vi "IDS Set Get ROI.vi"(0 "IDS Notifier Ref":refnum<notifier>, 5 "IDS Actions":T1, 7 "IDS Camera Ref":refnum<k24>, 9 "IDS Image Ref":T2, 11 "Error":errorcluster) -> (4 "IDS Notifier Ref (Dup)":refnum<notifier>, 15 "Error":errorcluster)   [LabVIEW 2025]
uses:
  C:/Users/Photonics03/Documents/Microscope-Control/Device Library/Cameras/IDS/IDS LabView Examples/LabVIEW/ueye.NET/uEyeDotNet.dll
  IDS LabView Examples/LabVIEW/ueye.NET/uEyeDotNet.dll
  <vilib>/vision/Image Controls.llb/IMAQ Image.ctl
  IDS Controls/IDS Notifier Element.ctl
  IDS Controls/IDS Actions.ctl
  IDS Controls/IDS Parameters.ctl
  IDS Controls/IDS Parameter List.ctl
  IDS Controls/IDS ROI.ctl
  Camera Controls/Camera IMAQ Key Info.ctl
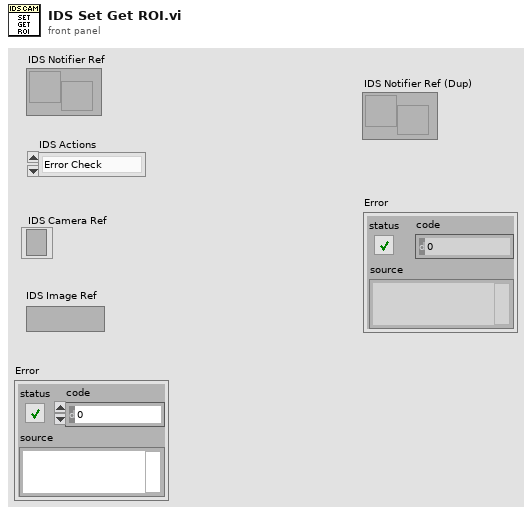
[diagram p1: front panel]
types:
  T1 = typedef "IDS Actions.ctl" = enum16{"Error Check", "Initialize", "Preview", "Record", "Abort", "Record Settings", "Set Parameter", "Get Parameter", "Set ROI", "Get ROI", "Status", "Quit"}
  T2 = typedef "IMAQ Image.ctl" = refnum<image>
  T3 = typedef "Camera IMAQ Key Info.ctl" = cluster{"Frame":u32, "Sensor Height":i32, "Sensor Width":i32, "ROI Height":i32, "ROI Width":i32, "ROI Enable?":bool, "Bit per Pixel":u8}
  T4 = typedef "IDS Notifier Element.ctl" = cluster{"IDS Actions":T1, "Received?":bool, "IDS Parameter":T5, "IDS ROI":T7, "Running?":bool, "File Path":path, "# of frames":u32, "Image Ref":T2, "Error":errorcluster, "Binning":i32}
  T5 = typedef "IDS Parameters.ctl" = cluster{"Parameter":T6, "Value":dbl}
  T6 = typedef "IDS Parameter List.ctl" = enum16{"Exposure Time (s)", "Binning"}
  T7 = typedef "IDS ROI.ctl" = cluster{"H Offset":i32, "V Offset":i32, "H Width":i32, "V Width":i32}
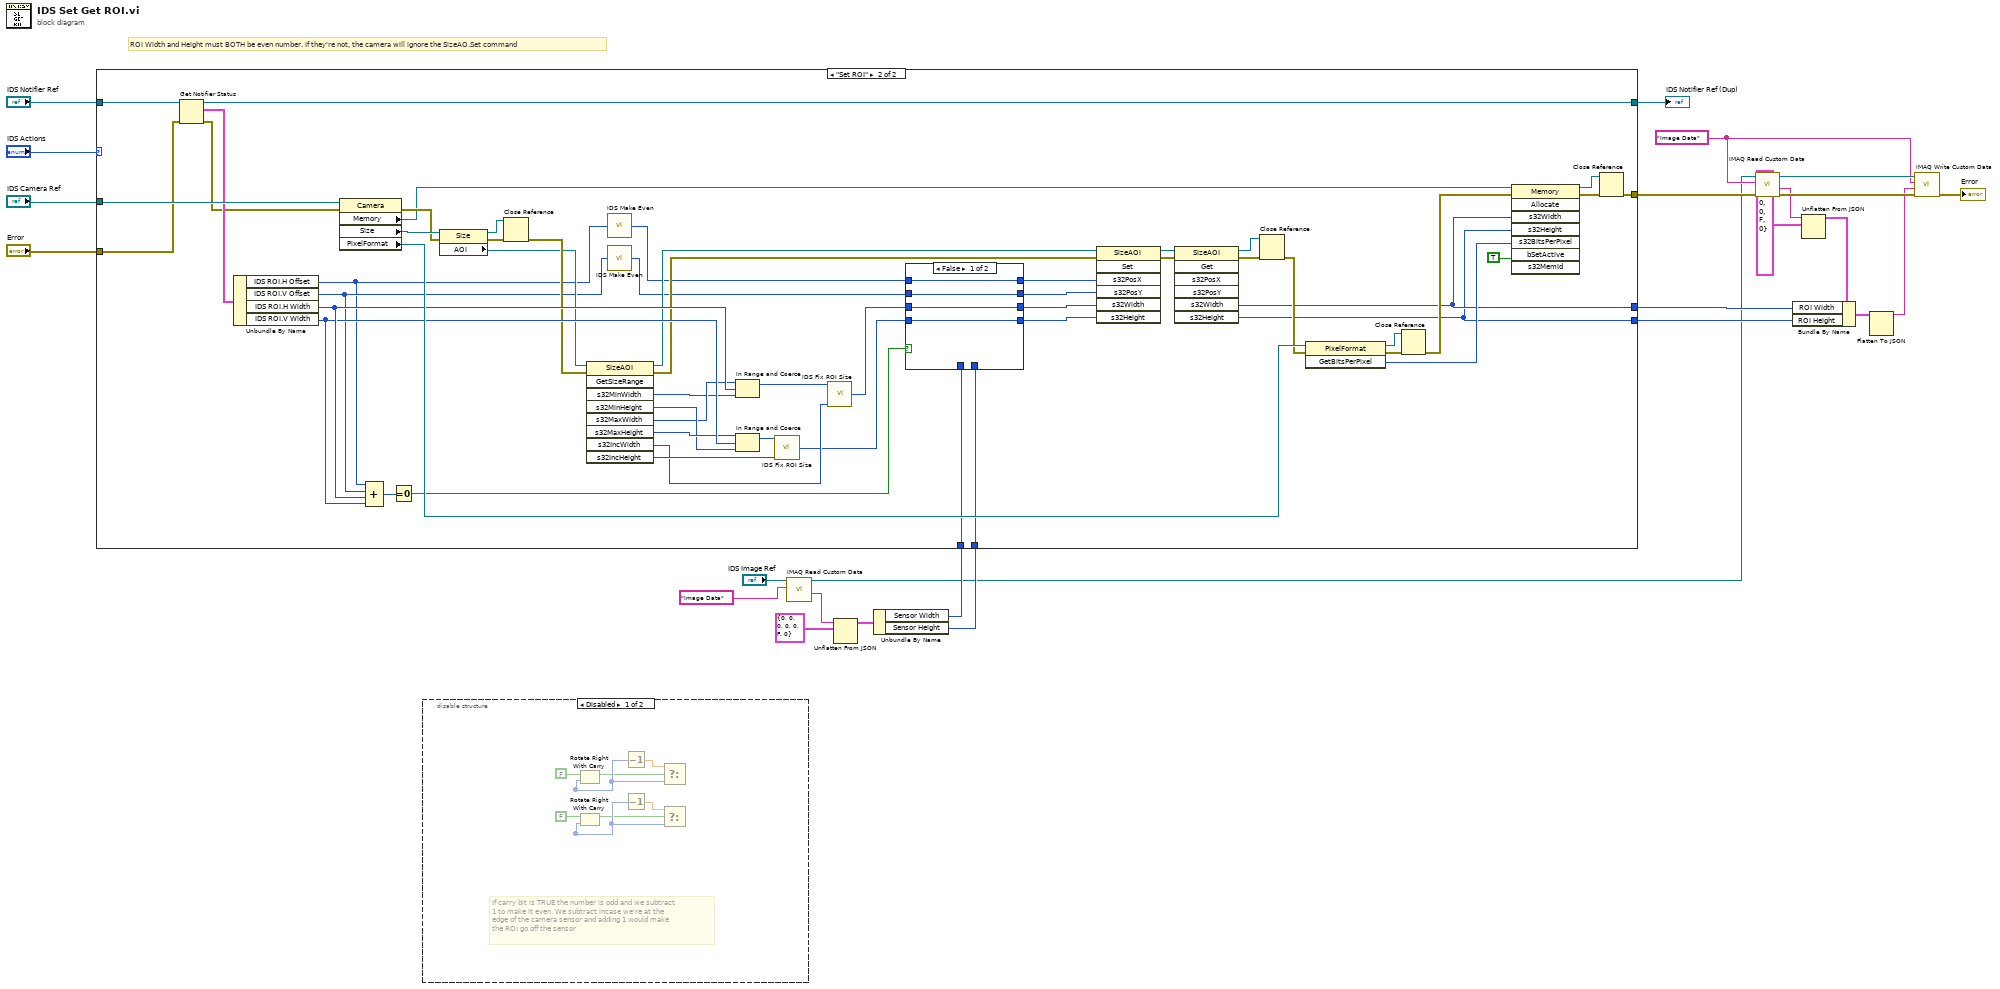
[diagram p0: block diagram]
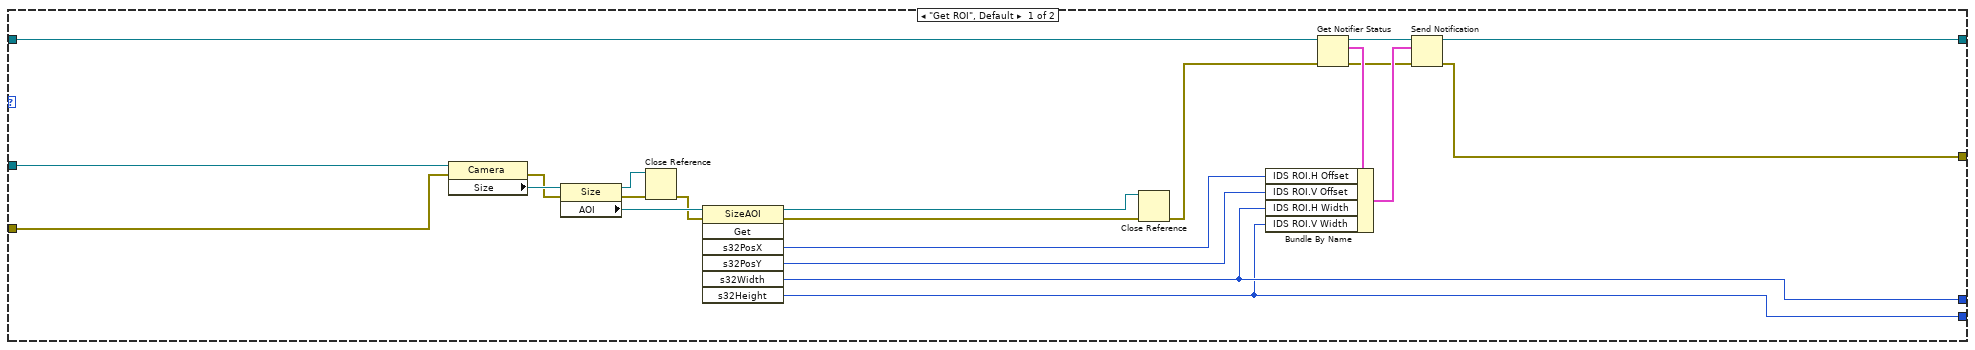
[diagram p3: hidden frame]
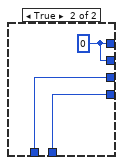
[diagram p4: hidden frame]
diagram:
  w13 = "Image Data" ("Key")
  # "ROI Width and Height must BOTH be even number. If they're not, the camera will ignore the SizeAO.Set command"
  n1 = disable-structure shown="Disabled" {
    frame Disabled {
      # "If carry bit is TRUE the number is odd and we subtract\n1 to make it even. We subtract incase we're at the\nedge of the camera sensor and adding 1 would make\nthe ROI go off the sensor"
      n2 = Rotate Right With Carry(3:FALSE ("carry")) -> (1:w29:bool, 2:w33:i32)  [unwired: 1 out]
      n3 = Rotate Right With Carry(3:FALSE ("carry")) -> (1:w28:bool, 2:w31:i32)  [unwired: 1 out]
      n4 = Decrement(x=w33) -> (x-1=w30:dbl)
      n5 = Decrement(x=w31) -> (x-1=w32:dbl)
      n6 = Select(t=w30, s=w29, f=w33) -> ()  [unwired: 1 out]
      n7 = Select(t=w32, s=w28, f=w31) -> ()  [unwired: 1 out]
    }
    frame Enabled {
    }
  }
  n8 = call "IMAQ Read Custom Data"("Key"="Image Data", "Image"="IDS Image Ref") -> ("Custom Data Out"=w7:string, "Image (duplicate)"=w2:T2)  [unwired: 7 in, 1 out]
  n9 = Unflatten From JSON(JSON string=w7, type and defaults=T3 {"Frame"=0, "Sensor Height"=0, "Sensor Width"=0, "ROI Height"=0, "ROI Width"=0, "ROI Enable?"=FALSE, "Bit per Pixel"=0} ("Camera IMAQ Key Info")) -> (value=w6:T3)  [unwired: 5 in, 1 out]
  n10 = Unbundle By Name(w6) -> ("Sensor Width"=w5:i32, "Sensor Height"=w4:i32)
  n11 = case shown="\"Set ROI\"" "IDS Actions" {
    tunnel: "IDS Camera Ref" -> [w48 w101]
    tunnel: "Error" -> [w45 w88]
    tunnel: "IDS Notifier Ref" -> [w47 w92]
    tunnel: [w35 w91] -> w21
    tunnel: [w36 w86] -> w11
    tunnel: [w40 w85] -> w10
    tunnel: [w39 w84] -> w9
    tunnel: w5 -> [_ w60]
    tunnel: w4 -> [_ w61]
    frame "Get ROI", Default {
      n12 = property class="Camera"(reference=w48, error in=w45) -> (error out=w54:errorcluster, "Size"=w55:refnum<k24>)  [unwired: 1 out]
      n13 = property class="Size"(reference=w55, error in=w54) -> (reference out=w52:refnum<k24>, error out=w53:errorcluster, "AOI"=w51:refnum<k24>)
      n14 = Close Reference(reference=w52, error in (no error)=w53) -> (error out=w49:errorcluster)
      n15 = invoke class="SizeAOI" method="Get"(reference=w51, error in=w49) -> (reference out=w34:refnum<k24>, error out=w50:errorcluster, "s32PosX"=w42:i32, "s32PosY"=w41:i32, "s32Width"=w40:i32, "s32Height"=w39:i32)  [unwired: 5 in, 1 out]
      n16 = Close Reference(reference=w34, error in (no error)=w50) -> (error out=w44:errorcluster)
      n17 = Get Notifier Status(notifier=w47, error in (no error)=w44) -> (notifier out=w46:refnum<notifier>, current notification=w43:T4, error out=w37:errorcluster)  [unwired: 2 out]
      n18 = Bundle By Name(cluster=w43, "IDS ROI.H Offset"=w42, "IDS ROI.V Offset"=w41, "IDS ROI.H Width"=w40, "IDS ROI.V Width"=w39) -> (w38:T4)
      n19 = Send Notification(notification=w38, notifier=w46, error in (no error)=w37) -> (notifier out=w35:refnum<notifier>, error out=w36:errorcluster)
    }
    frame "Set ROI" {
      n20 = Get Notifier Status(notifier=w92, error in (no error)=w88) -> (notifier out=w91:refnum<notifier>, current notification=w90:T4, error out=w87:errorcluster)  [unwired: 2 out]
      n21 = Unbundle By Name(w90) -> ("IDS ROI.H Offset"=w57:i32, "IDS ROI.V Offset"=w59:i32, "IDS ROI.H Width"=w82:i32, "IDS ROI.V Width"=w81:i32)
      n22 = property class="Camera"(reference=w101, error in=w87) -> (error out=w97:errorcluster, "Memory"=w89:refnum<k24>, "Size"=w110:refnum<k24>, "PixelFormat"=w109:refnum<k24>)  [unwired: 1 out]
      n23 = Compound Arithmetic op=ADD(w57, w59, w82, w81) -> (w83:i32)
      n24 = Equal To 0?(x=w83) -> (x = 0?=w62:bool)
      n25 = property class="Size"(reference=w110, error in=w97) -> (reference out=w104:refnum<k24>, error out=w100:errorcluster, "AOI"=w75:refnum<k24>)
      n26 = Close Reference(reference=w104, error in (no error)=w100) -> (error out=w76:errorcluster)
      n27 = invoke class="SizeAOI" method="GetSizeRange"(reference=w75, error in=w76) -> (reference out=w74:refnum<k24>, error out=w73:errorcluster, "s32MinWidth"=w77:i32, "s32MinHeight"=w79:i32, "s32MaxWidth"=w78:i32, "s32MaxHeight"=w80:i32, "s32IncWidth"=w69:i32, "s32IncHeight"=w70:i32)  [unwired: 7 in, 1 out]
      n28 = call "IDS Make Even.vi"("Input"=w57) -> ("Even Output"=w56:i32)  [unwired: 14 in]
      n29 = call "IDS Make Even.vi"("Input"=w59) -> ("Even Output"=w58:i32)  [unwired: 14 in]
      n30 = In Range and Coerce(upper limit=w78, x=w82, lower limit=w77) -> (coerced(x)=w72:i32)  [unwired: 1 out]
      n31 = In Range and Coerce(upper limit=w80, x=w81, lower limit=w79) -> (coerced(x)=w71:i32)  [unwired: 1 out]
      n32 = call "IDS Fix ROI Size.vi"("Requested Value"=w71, "Allowed Increment"=w70) -> ("Resulting Value"=w67:i32)  [unwired: 13 in]
      n33 = call "IDS Fix ROI Size.vi"("Requested Value"=w72, "Allowed Increment"=w69) -> ("Resulting Value"=w68:i32)  [unwired: 13 in]
      n34 = case shown="False" w62 {
        tunnel: [w114 w117] -> w63
        tunnel: w56 -> [w114 _]
        tunnel: [w113 w117] -> w64
        tunnel: w58 -> [w113 _]
        tunnel: [w112 w115] -> w65
        tunnel: w68 -> [w112 _]
        tunnel: [w111 w116] -> w66
        tunnel: w67 -> [w111 _]
        tunnel: w61 -> [_ w116]
        tunnel: w60 -> [_ w115]
        frame False {
        }
        frame True {
          w117 = 0 ("H Offset")
        }
      }
      n35 = invoke class="SizeAOI" method="Set"(reference=w74, error in=w73, "s32PosX"=w63, "s32PosY"=w64, "s32Width"=w65, "s32Height"=w66) -> (reference out=w106:refnum<k24>, error out=w99:errorcluster)  [unwired: 1 in, 5 out]
      n36 = invoke class="SizeAOI" method="Get"(reference=w106, error in=w99) -> (reference out=w102:refnum<k24>, error out=w98:errorcluster, "s32Width"=w85:i32, "s32Height"=w84:i32)  [unwired: 5 in, 3 out]
      n37 = Close Reference(reference=w102, error in (no error)=w98) -> (error out=w96:errorcluster)
      n38 = invoke class="PixelFormat" method="GetBitsPerPixel"(reference=w109, error in=w96) -> (reference out=w105:refnum<k24>, error out=w95:errorcluster, "GetBitsPerPixel"=w107:i32)  [unwired: 1 in]
      n39 = Close Reference(reference=w105, error in (no error)=w95) -> (error out=w94:errorcluster)
      n40 = invoke class="Memory" method="Allocate"(reference=w89, error in=w94, "s32Width"=w85, "s32Height"=w84, "s32BitsPerPixel"=w107, "bSetActive"=TRUE) -> (reference out=w103:refnum<k24>, error out=w93:errorcluster)  [unwired: 2 in, 6 out]
      n41 = Close Reference(reference=w103, error in (no error)=w93) -> (error out=w86:errorcluster)
    }
  }
  "IDS Notifier Ref (Dup)" <- w21
  n42 = call "IMAQ Read Custom Data"("error in (no error)"=w11, "Key"=w13, "Image"=w2) -> ("error out"=w20:errorcluster, "Custom Data Out"=w16:string, "Image (duplicate)"=w15:T2)  [unwired: 6 in]
  n43 = Unflatten From JSON(JSON string=w16, type and defaults=T3 {"Frame"=0, "Sensor Height"=0, "Sensor Width"=0, "ROI Height"=0, "ROI Width"=0, "ROI Enable?"=FALSE, "Bit per Pixel"=0} ("Camera IMAQ Key Info")) -> (value=w17:T3)  [unwired: 5 in, 1 out]
  n44 = Bundle By Name(cluster=w17, "ROI Width"=w10, "ROI Height"=w9) -> (w18:T3)
  n45 = Flatten To JSON(anything=w18) -> (JSON string=w19:string)  [unwired: 2 in, 1 out]
  n46 = call "IMAQ Write Custom Data"("error in (no error)"=w20, "Custom Data In"=w19, "Key"=w13, "Image"=w15) -> ("error out"=→"Error":errorcluster)  [unwired: 6 in, 1 out]
